vi "Message handle.vi"(0 "queue in":refnum<queue>, 5 "Command":T1=enum."MCU Reset", 7 "DATA[X]":u8[](array[numeric]), 11 "error in (no error)":errorcluster) -> (4 "Communication":T2(array[cluster]) {"ID" format="%.0x"; "DATA[0]" format="%.0x"; "DATA[1]" format="%.0x"; "DATA[2]" format="%.0x"; "DATA[3]" format="%.0x"; "DATA[4]" format="%.0x"; "DATA[5]" format="%.0x"; "DATA[6]" format="%.0x"; "DATA[7]" format="%.0x"}, 6 "Correct answer":bool, 8 "String test data":string, 10 "Numeric test data":sgl[](array[numeric]), 14 "timed out?":bool, 15 "error out":errorcluster)   [LabVIEW 2025]
uses:
  Controls/CAN Sending Data.ctl
  Controls/CAN Payload.ctl
  Commands.ctl
  Notifier Data.ctl
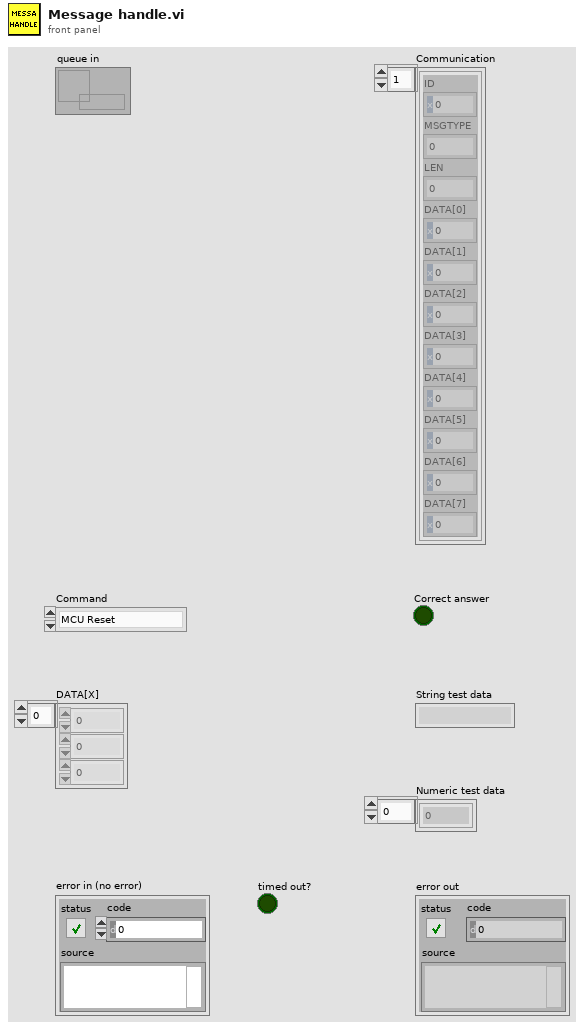
[diagram p1: front panel]
types:
  T1 = typedef "Commands.ctl" = enum16{"Nexteer connect", "Write Polarity", "Write BEMF", "Write Torque Scale Sensors T1", "Write Torque Scale Sensors T2", "Trim HW Torque Sensors T1", "Trim HW Torque Sensors T2", "Read HW Torque Trim Performed Sensors T1", "Read HW Torque Trim Performed Sensors T2", "Write EOL Offset values to defaults", "Write EOL Gain values to defaults", "Write Serial Number", "Write Hardware Part Number", "Write EPS Serial Number", "Read MEC Counter", "MCU Reset", "Read System State", "Read First Motor Position", "Manufacturing Diagnostic Defeat", "Perform Current Offset ", "Current Offset Status", "Enable Engine Run", "Perform Current Gain ", "Current Gain Status", "Disable Torque Ramp Down ", "Disable Engine Run", "Set Vehicle Speed Override", "Read Offset Values Using FD F5", "Read Gain Values Using FD F4", "Clear Nexteer NTCs", "Read Second Motor Position", "Read ECU Software ID", "Read Internal Software Version", "Read Bootloader ID", "Read Bootloader Software Version", "Read Calibration Release 0", "Read Calibration Release 1", "Read Calibration Release 2", "Read Temperature  ", "Battery Voltage  ", "Read Motor Angle 0", "Read Motor Angle 1 ", "Set Motor Torque Command ", "Read Motor Current   ", "Stop Motor Torque Command", "Read NTCs", "Read Serial Number", "Read HW Part Number", "Read Polarity", "Set NVM Access Defeat", "Read Software Release", "Read Software Build Date", "Write Single Inverter Hardware value", "Write Dual Inverter Hardware value", "Read Single Inverter HW Value", "Read Dual Inverter HW Value", "Write MEC Counter FE", "Write MEC Counter FF", "Read BEMF", "Read Torque 1 FDB6", "Read Torque 2 FDB7", "Read Torque Trim 1 FDB4", "Read Torque Trim 2 FDB5", "Write Torque Trim 1 FDB4", "Write Torque Trim 2 FDB5", "XCP connect", "Read HW Torque T1", "Read HW Torque T2", "Read Motor Speed "}
  T2 = cluster{"ID":u32, "MSGTYPE":u8, "LEN":u8, "DATA[0]":u8, "DATA[1]":u8, "DATA[2]":u8, "DATA[3]":u8, "DATA[4]":u8, "DATA[5]":u8, "DATA[6]":u8, "DATA[7]":u8}[]
  T3 = typedef "CAN Sending Data.ctl" = cluster{"Channel reference":u16, "MessagesToSend":cluster{"ID":u32, "MSGTYPE":u8, "LEN":u8, "DATA[0]":u8, "DATA[1]":u8, "DATA[2]":u8, "DATA[3]":u8, "DATA[4]":u8, "DATA[5]":u8, "DATA[6]":u8, "DATA[7]":u8}, "NoMessages":i32[], "Nexteer/XCP?":bool, "CAN Payload Array":T4[], "Expected responses":cluster{"DATA[0]":u8, "DATA[1]":u8, "DATA[2]":u8, "DATA[3]":u8}[], "Command":T1, "DATA[X]":u8[], "notifier out":refnum<notifier>}
  T4 = typedef "CAN Payload.ctl" = cluster{"DATA[0]":u8, "DATA[1]":u8, "DATA[2]":u8, "DATA[3]":u8, "DATA[4]":u8, "DATA[5]":u8, "DATA[6]":u8, "DATA[7]":u8}
  T5 = typedef "Notifier Data.ctl" = cluster{"Communication":cluster{"ID":u32, "MSGTYPE":u8, "LEN":u8, "DATA[0]":u8, "DATA[1]":u8, "DATA[2]":u8, "DATA[3]":u8, "DATA[4]":u8, "DATA[5]":u8, "DATA[6]":u8, "DATA[7]":u8}[], "Correct answer":bool}
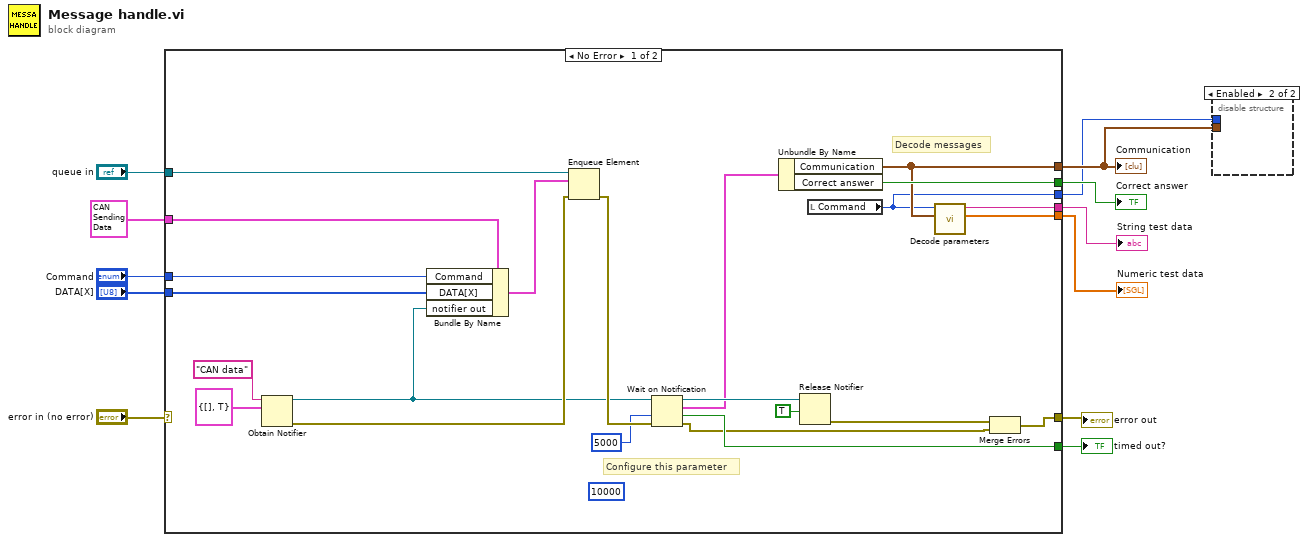
[diagram p0: block diagram]
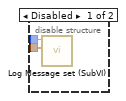
[diagram p2: hidden frame]
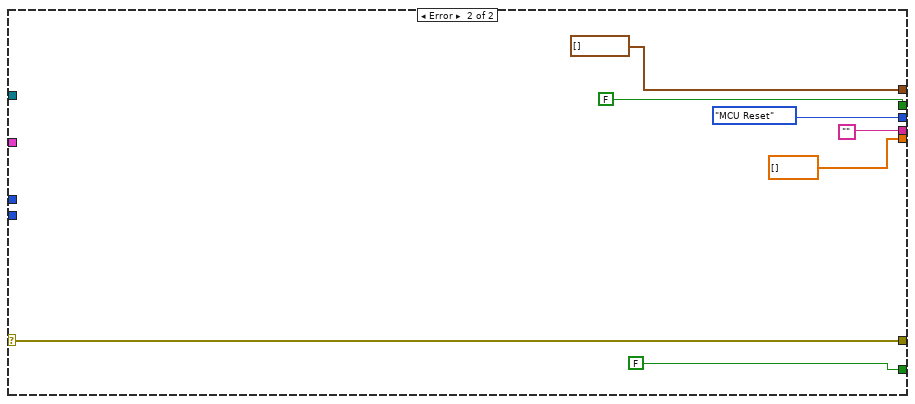
[diagram p3: hidden frame]
diagram:
  n1 = case shown="No Error" "error in (no error)" {
    selector: "error in (no error)" -> [_ w42]
    tunnel: T3 {"Channel reference"=0, "MessagesToSend"={"ID"=0, "MSGTYPE"=0, "LEN"=0, "DATA[0]"=0, "DATA[1]"=0, "DATA[2]"=0, "DATA[3]"=0, "DATA[4]"=0, "DATA[5]"=0, "DATA[6]"=0, "DATA[7]"=0}, "NoMessages"=[], "Nexteer/XCP?"=FALSE, "CAN Payload Array"=[], "Expected responses"=[], "Command"=enum."MCU Reset", "DATA[X]"=[], "notifier out"=refnum} -> [w35 _]
    tunnel: [w28 w42] -> w11
    tunnel: [w27 FALSE ("timed out?")] -> w10
    tunnel: "queue in" -> [w25 _]
    tunnel: [w23 FALSE ("Correct answer")] -> w7
    tunnel: [w19 ""] -> w6
    tunnel: [w18 sgl[] [] ("Numeric results")] -> w5
    tunnel: "Command" -> [w22 _]
    tunnel: "DATA[X]" -> [w21 _]
    tunnel: [w20 T2 [] ("Communication")] -> w2
    tunnel: [w13 Commands."MCU Reset" ("Command")] -> w1
    frame No Error {
      (unwired) 10000 ("timeout in ms (-1)")
      # "Decode messages"
      # "Configure this parameter"
      n2 = Obtain Notifier(name (unnamed)="CAN data", notification data type=T5 {"Communication"=[], "Correct answer"=TRUE}) -> (notifier out=w16:refnum<notifier>, error out=w33:errorcluster)  [unwired: 2 in, 1 out]
      n3 = Bundle By Name(cluster=w35, "Command"=w22, "DATA[X]"=w21, "notifier out"=w16) -> (w24:T3)
      n4 = Enqueue Element(queue=w25, element=w24, error in (no error)=w33) -> (error out=w34:errorcluster)  [unwired: 1 in, 2 out]
      n5 = Wait on Notification(notifier=w16, timeout in ms (-1)=5000, error in (no error)=w34) -> (notifier out=w32:refnum<notifier>, notification=w30:T5, timed out?=w27:bool, error out=w14:errorcluster)  [unwired: 1 in]
      n6 = Unbundle By Name(w30) -> ("Communication"=w20:T2, "Correct answer"=w23:bool)
      n7 = Release Notifier(notifier=w32, force destroy? (F)=TRUE) -> (error out=w29:errorcluster)  [unwired: 1 in, 2 out]
      n8 = local read "Command"() -> (w13:T1)
      n9 = call "Decode parameters.vi"("Comminication in"=w20, "Commands"=w13) -> ("Numeric results"=w18:sgl[], "String results"=w19:string)  [unwired: 8 in]
      n10 = Merge Errors(w29, w14) -> (w28:errorcluster)
    }
    frame Error {
    }
  }
  "error out" <- w11
  "timed out?" <- w10
  "Communication" <- w2
  "Correct answer" <- w7
  "String test data" <- w6
  "Numeric test data" <- w5
  n11 = disable-structure shown="Enabled" {
    disable-tunnel: w2 -> [w44 _]
    disable-tunnel: w1 -> [w43 _]
    frame Disabled {
      n12 = call "Log Message set (SubVI).vi"("Communication"=w44, "Command"=w43) -> ()  [unwired: 10 in]
    }
    frame Enabled {
    }
  }
